vi "HXG2_TableFormatting.vi"(8 "error IO":errorcluster, 9 "Programmer File":string, 10 "Data Array In":string[][](array[string]), 11 "Table Control":refnum<vi>) -> (0 "error out":errorcluster, 3 "Headers":string[][](array[string]))   [LabVIEW 2012]
doc: "On the programmer table setup all headers (constants) and setup formatting"
uses:
  <vilib>/Utility/miscctls.llb/LVRowAndColumnTypeDef.ctl
  <vilib>/Utility/miscctls.llb/LVBoundsTypeDef.ctl
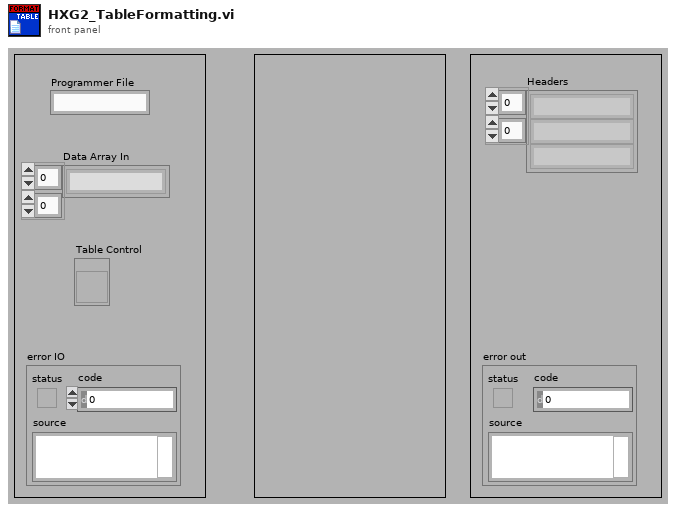
[diagram p1: front panel]
types:
  T1 = typedef "LVBoundsTypeDef.ctl" = cluster{"Width":u32, "Height":u32}
  T2 = typedef "LVRowAndColumnTypeDef.ctl" = cluster{"Row":i32, "Column":i32}
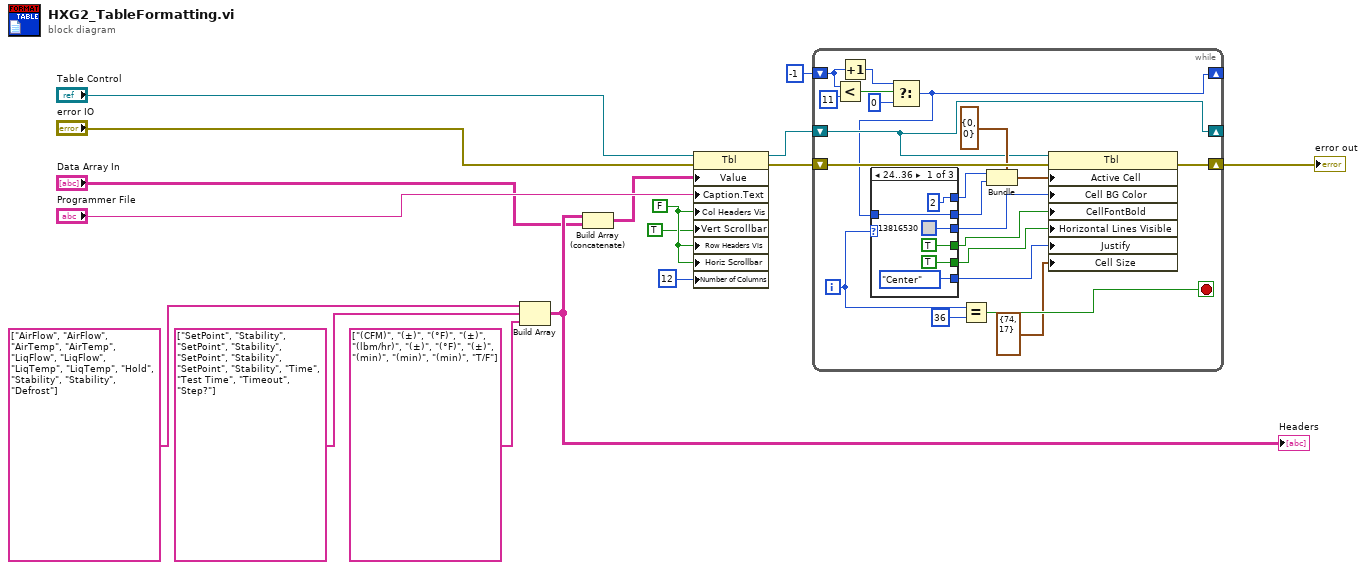
[diagram p0: block diagram]
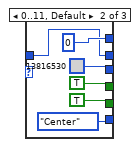
[diagram p2: hidden frame]
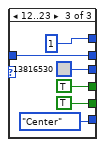
[diagram p3: hidden frame]
diagram:
  w16 = FALSE ("Visible Items:Column Headers Visible")
  n1 = Build Array(string[] ["AirFlow", "AirFlow", "AirTemp", "AirTemp", "LiqFlow", "LiqFlow", "LiqTemp", "LiqTemp", "Hold", "Stability", "Stability", "Defrost"], string[] ["SetPoint", "Stability", "SetPoint", "Stability", "SetPoint", "Stability", "SetPoint", "Stability", "Time", "Test Time", "Timeout", "Step?"], string[] ["(CFM)", "(±)", "(°F)", "(±)", "(lbm/hr)", "(±)", "(°F)", "(±)", "(min)", "(min)", "(min)", "T/F"]) -> (w4:string[][])
  "Headers" <- w4
  n2 = Build Array (concatenate)(w4, "Data Array In") -> (w2:string[][])
  n3 = property class="Tbl"(reference="Table Control", error in="error IO", "Value"=w2, "Caption.Text"="Programmer File", "Col Headers Vis"=w16, "Vert Scrollbar"=TRUE ("Visible Items:Vertical Scrollbar Visible"), "Row Headers Vis"=w16, "Horiz Scrollbar"=w16, "Number of Columns"=u32 12) -> (reference out=w11:refnum<vi>, error out=w12:errorcluster)
  n4 = while {
    shift-right: [w24] -> _
    shift-left: -1 ("f") -> [w28]
    shift-right: [w37] -> w13
    shift-left: w12 -> [w36]
    shift-right: [w25] -> _
    shift-left: w11 -> [w25]
    i -> [w32]
    stop <- w35 stop-if-true
    n5 = Less?(x=w28, y=11) -> (x < y?=w29:bool)
    n6 = Increment(x=w28) -> (x+1=w26:i32)
    n7 = Select(t=w26, s=w29, f=0) -> (s? t:f=w24:i32)
    n8 = case shown="24..36" w32 {
      tunnel: [w42 w44 w54] -> w31
      tunnel: [2 0 1] -> w30
      tunnel: w24 -> [w42 w44 w54]
      tunnel: [u32 13816530 u32 13816530 u32 13816530] -> w21
      tunnel: [TRUE ("Active Cell:Cell Font:Bold") TRUE ("Active Cell:Cell Font:Bold") TRUE ("Active Cell:Cell Font:Bold")] -> w20
      tunnel: [TRUE ("Active Cell:Cell Font:Bold") TRUE ("Active Cell:Cell Font:Bold") TRUE ("Active Cell:Cell Font:Bold")] -> w19
      tunnel: [enum16{"Left", "Center", "Right"}."Center" ("Active Cell:Cell Justification") enum16{"Left", "Center", "Right"}."Center" ("Active Cell:Cell Justification") enum16{"Left", "Center", "Right"}."Center" ("Active Cell:Cell Justification")] -> w17
      frame 24..36 {
      }
      frame 0..11, Default {
      }
      frame 12..23 {
      }
    }
    n9 = Equal?(x=w32, y=36) -> (x = y?=w35:bool)
    n10 = Bundle(cluster=T2 {"Row"=0, "Column"=0} ("Active Cell:Active Cell"), "Row"=w30, "Column"=w31) -> (w34:T2)
    n11 = property class="Tbl"(reference=w25, error in=w36, "Active Cell"=w34, "Cell BG Color"=w21, "CellFontBold"=w20, "Horizontal Lines Visible"=w19, "Justify"=w17, "Cell Size"=T1 {"Width"=74, "Height"=17} ("Active Cell:Cell Size")) -> (error out=w37:errorcluster)  [unwired: 1 out]
  }
  "error out" <- w13
